vi "GetSingleInstrument.vi"(8 "error in (no error)":errorcluster, 10 "ID":string, 11 "ByteGSWebAPI-V0 in":refnum<class "ByteGSWebAPI-V0.lvclass">) -> (0 "error out":errorcluster, 2 "InstrumentData":T1, 3 "ByteGSWebAPI-V0 out":refnum<class "ByteGSWebAPI-V0.lvclass">, 4 "body":string, 6 "headers":string)   [LabVIEW 2019, in "ByteGSWebAPI.lvlib" / "ByteGSWebAPI-V0.lvclass"]
uses:
  ByteGSWebAPI-V0.lvclass
  Cntrls/SingleInstrument.ctl
  cafd0801-0ee5-4417-b853-6a6d16c7dcb3.vi
  <vilib>/JDP Science/JSONtext/JSON text to Variant.vi
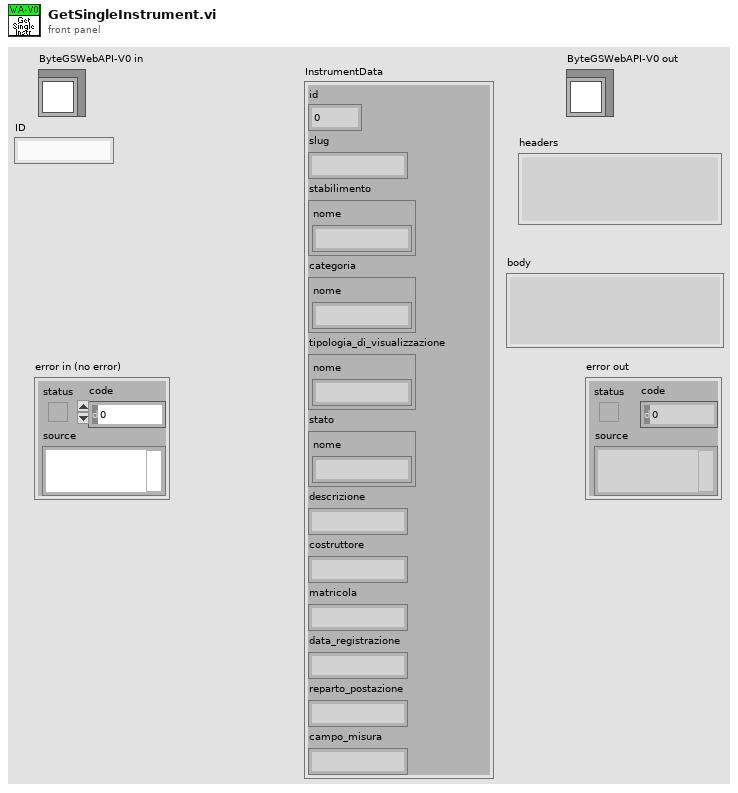
[diagram p1: front panel]
types:
  T1 = typedef "ByteGSWebAPI.lvlib/ByteGSWebAPI-V0.lvclass/SingleInstrument.ctl" = cluster{"id":i32, "slug":string, "stabilimento":cluster{"nome":string}, "categoria":cluster{"nome":string}, "tipologia_di_visualizzazione":cluster{"nome":string}, "stato":cluster{"nome":string}, "descrizione":string, "costruttore":string, "matricola":string, "data_registrazione":string, "reparto_postazione":string, "campo_misura":string}
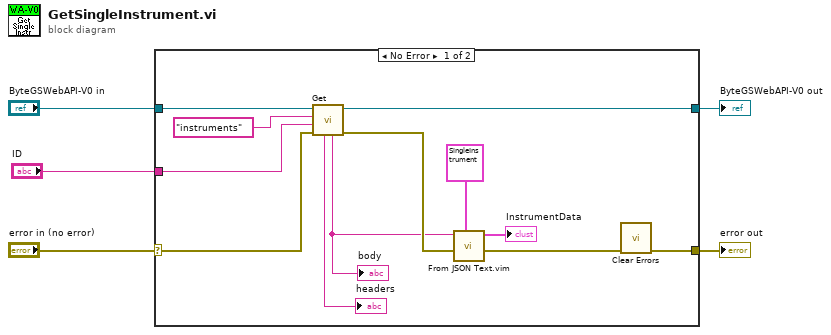
[diagram p0: block diagram]
diagram:
  n1 = case shown="No Error" "error in (no error)" {
    selector: "error in (no error)" -> [w15 w19]
    tunnel: [w9 w19] -> w4
    tunnel: [w14 w18] -> w2
    tunnel: "ByteGSWebAPI-V0 in" -> [w17 w18]
    tunnel: "ID" -> [w12 _]
    frame No Error {
      n2 = call-dynamic "Get.vi"("error in (no error)"=w15, "Parameter"=w12, "Request"="instruments" ("Parameter"), "ByteGSWebAPI-V0 in"=w17) -> ("error out"=w11:errorcluster, "ByteGSWebAPI-V0 out"=w14:refnum<class "ByteGSWebAPI-V0.lvclass">, "body"=w8:string, "headers"=→"headers":string)  [unwired: 4 in]
      "body" <- w8
      n3 = call "From JSON Text.vim"("Data Type and Default Value"=T1 {"id"=0, "slug"="", "stabilimento"={"nome"=""}, "categoria"={"nome"=""}, "tipologia_di_visualizzazione"={"nome"=""}, "stato"={"nome"=""}, "descrizione"="", "costruttore"="", "matricola"="", "data_registrazione"="", "reparto_postazione"="", "campo_misura"=""} ("SingleInstrument"), "error in (no error)"=w11, "JSON"=w8) -> ("error out"=w10:errorcluster, "Data out"=→"InstrumentData":T1)  [unwired: 7 in]
      n4 = call <vilib>:"Clear Errors.vi"("error in (no error)"=w10) -> ("error out"=w9:errorcluster)  [unwired: 5 in, 1 out]
    }
    frame Error {
    }
  }
  "error out" <- w4
  "ByteGSWebAPI-V0 out" <- w2
